vi "niFpga wdp fft input buffer dummy.vi"(4 "enable":bool, 6 "write memory 2?":bool, 8 "read index":fxp<+,9,9>, 9 "write index":fxp<+,8,8>, 10 "data in im":fxp<+/-,8,1>[](array[numeric])=[0.0, 0.0], 11 "data in re":fxp<+/-,8,1>[](array[numeric])=[0.0, 0.0]) -> (2 "data out 1":T1, 3 "data out 0":T1)   [LabVIEW 2017]
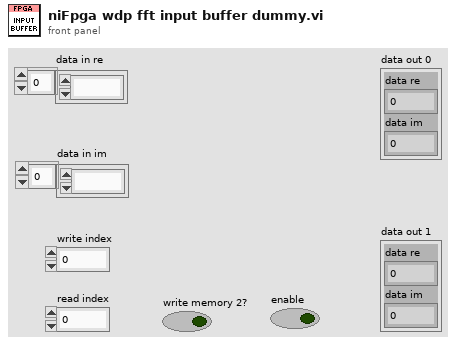
[diagram p1: front panel]
types:
  T1 = cluster{"internal input type":fxp<+/-,8,1>, "internal input type":fxp<+/-,8,1>}
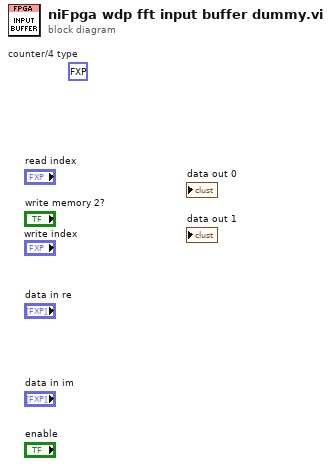
[diagram p0: block diagram]
diagram:
  (unwired) fxp<+,7,7> 0.0  # counter/4 type
